vi "Compare_Global_Values_Modify_Cost_f()-3.vi"(4 "[IN] Mean dR":dbl[](array[numeric]), 5 "error IN":errorcluster, 6 "[IN] Linearity":u8[](array[numeric]), 7 "[IN] Array of Mean\n(dR) - Problem dR":dbl[](array[numeric]), 8 "[IN] SD(Areas)":dbl[](array[numeric]), 9 "[IN] Array of Mean(Areas)\n - Problem finish Area":dbl[](array[numeric]), 10 "[IN] SD(dR)":dbl[](array[numeric]), 11 "[IN] Cost function":i8[](array[numeric])) -> (0 "error OUT":errorcluster, 3 "[OUT] Cost function":i8[](array[numeric]))   [LabVIEW 2013]
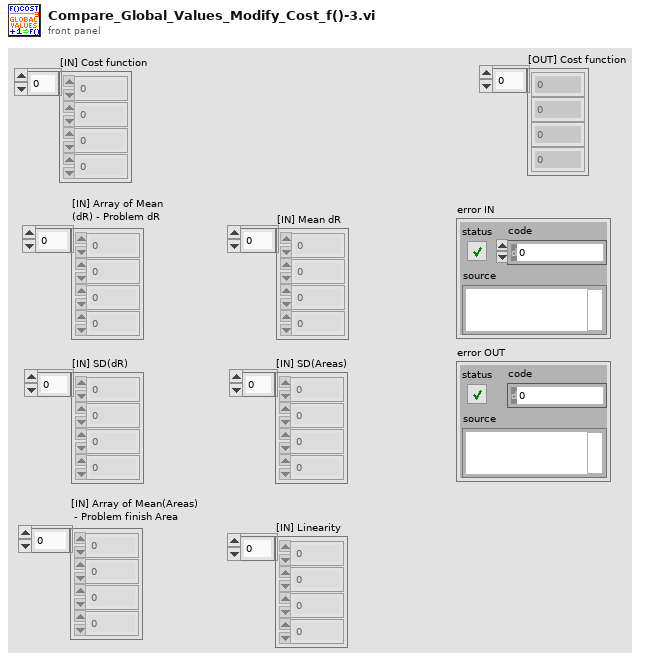
[diagram p1: front panel]
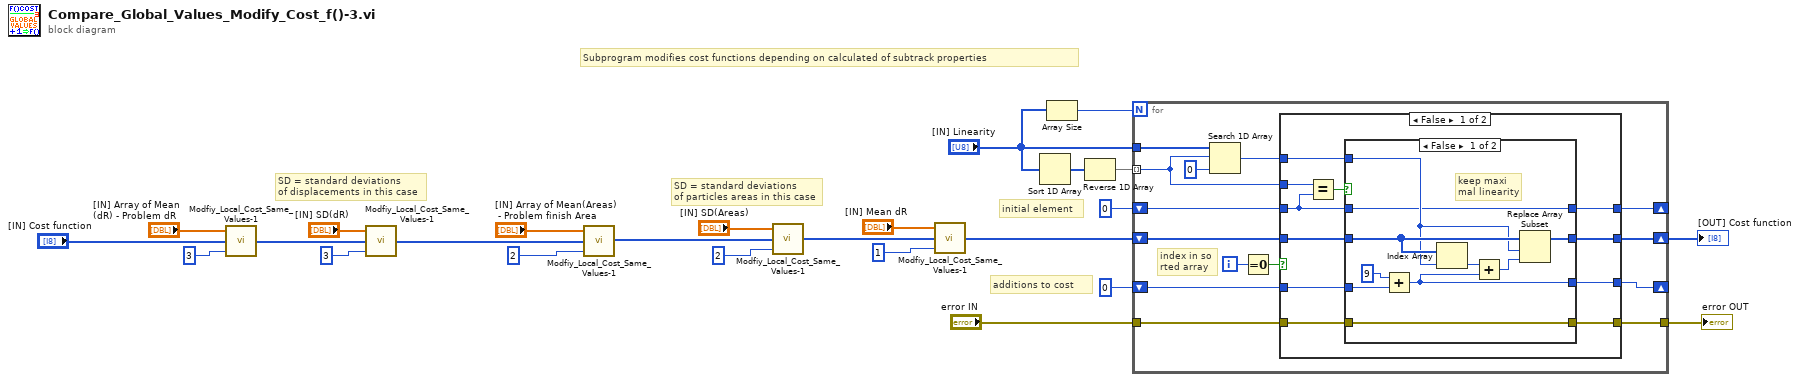
[diagram p0: block diagram]
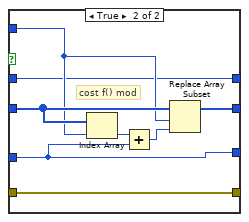
[diagram p2: hidden frame]
diagram:
  # "SD = standard deviations\nof particles areas in this case"
  # "SD = standard deviations\nof displacements in this case"
  # "additions to cost"
  # "initial element"
  # "Subprogram modifies cost functions depending on calculated of subtrack properties"
  n1 = call "Modfiy_Local_Cost_Same_Values-1.vi"("[IN] Cost Mutilplier"=i8 3, "[IN] Cost Function"="[IN] Cost function", "[IN] Array of Compared Values"="[IN] Array of Mean\n(dR) - Problem dR") -> ("[OUT] Cost Function"=w15:i8[])  [unwired: 2 in]
  n2 = call "Modfiy_Local_Cost_Same_Values-1.vi"("[IN] Cost Mutilplier"=i8 3 ("y"), "[IN] Cost Function"=w15, "[IN] Array of Compared Values"="[IN] SD(dR)") -> ("[OUT] Cost Function"=w13:i8[])  [unwired: 2 in]
  n3 = call "Modfiy_Local_Cost_Same_Values-1.vi"("[IN] Cost Mutilplier"=i8 2 ("y"), "[IN] Cost Function"=w13, "[IN] Array of Compared Values"="[IN] Array of Mean(Areas)\n - Problem finish Area") -> ("[OUT] Cost Function"=w9:i8[])  [unwired: 2 in]
  n4 = call "Modfiy_Local_Cost_Same_Values-1.vi"("[IN] Cost Mutilplier"=i8 2 ("y"), "[IN] Cost Function"=w9, "[IN] Array of Compared Values"="[IN] SD(Areas)") -> ("[OUT] Cost Function"=w3:i8[])  [unwired: 2 in]
  n5 = call "Modfiy_Local_Cost_Same_Values-1.vi"("[IN] Cost Mutilplier"=i8 1 ("y"), "[IN] Cost Function"=w3, "[IN] Array of Compared Values"="[IN] Mean dR") -> ("[OUT] Cost Function"=w2:i8[])  [unwired: 2 in]
  n6 = Sort 1D Array(array="[IN] Linearity") -> (sorted array=w25:u8[])
  n7 = Array Size(array="[IN] Linearity") -> (size(s)=w5:i32)
  n8 = Reverse 1D Array(array=w25) -> (reversed array=w24:u8[])
  n9 = for {
    N: w5 -> [_]
    tunnel: w24 -> [w35] mode=indexing
    tunnel: "[IN] Linearity" -> [w39]
    shift-right: [w33] -> w20
    shift-left: w2 -> [w34]
    shift-right: [w32] -> _
    shift-left: u8 0 -> [w31]
    shift-right: [w29] -> _
    shift-left: i8 0 -> [w30]
    tunnel: "error IN" -> [w27]
    tunnel: [w26] -> w21
    i -> [w37]
    # "index in so\nrted array"
    n10 = Search 1D Array(1D array=w39, element=w35, start index (0)=0) -> (index of element=w28:i32)
    n11 = Equal To 0?(x=w37) -> (x = 0?=w36:bool)
    n12 = case shown="False" w36 {
      tunnel: w35 -> [w46 w71]
      tunnel: [w45 w72] -> w33
      tunnel: w34 -> [w49 w72]
      tunnel: [w44 w71] -> w32
      tunnel: w31 -> [w40 _]
      tunnel: [w43 w70] -> w29
      tunnel: w30 -> [w47 w70]
      tunnel: w28 -> [w48 _]
      tunnel: w27 -> [w42 w69]
      tunnel: [w41 w69] -> w26
      frame False {
        n13 = Equal?(x=w46, y=w40) -> (x = y?=w50:bool)
        n14 = case shown="False" w50 {
          tunnel: w49 -> [w58 w66]
          tunnel: w48 -> [w55 w63]
          tunnel: w47 -> [w60 w65]
          tunnel: [w54 w64] -> w45
          tunnel: [w51 w61] -> w44
          tunnel: [w53 w65] -> w43
          tunnel: w42 -> [w52 w62]
          tunnel: [w52 w62] -> w41
          tunnel: w40 -> [w51 w61]
          frame False {
            # "keep maxi\nmal linearity"
            n15 = Add(x=i8 9 ("y"), y=w60) -> (x+y=w53:i8)
            n16 = Index Array(array=w58, index=w55) -> (element=w57:i8)
            n17 = Add(x=w57, y=w53) -> (x+y=w56:i8)
            n18 = Replace Array Subset(array=w58, new element=w56, index=w55) -> (w54:i8[])
          }
          frame True {
            # "cost f() mod"
            n19 = Index Array(array=w66, index=w63) -> (element=w67:i8)
            n20 = Add(x=w67, y=w65) -> (x+y=w68:i8)
            n21 = Replace Array Subset(array=w66, new element=w68, index=w63) -> (w64:i8[])
          }
        }
      }
      frame True {
        # "maximal linearity (!)"
      }
    }
  }
  "[OUT] Cost function" <- w20
  "error OUT" <- w21
